vi "tm_sensorcooler_40.vi"(8 "error in (no error)":errorcluster, 10 "Mode":i32(ring)=1 items=["Disable"=1, "Enable"=2], 11 "Handle in":u32) -> (0 "error out":errorcluster, 3 "Handle out":u32)   [LabVIEW 2023]
uses:
  tmcamcon.dll
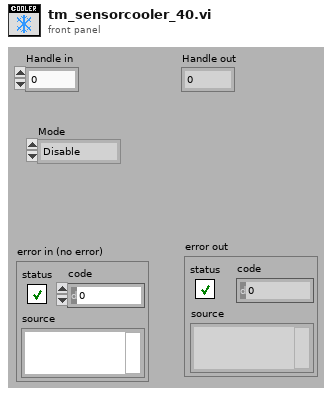
[diagram p1: front panel]
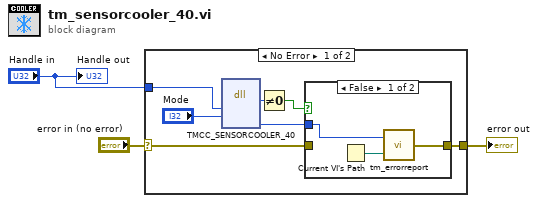
[diagram p0: block diagram]
diagram:
  n1 = case shown="No Error" "error in (no error)" {
    selector: "error in (no error)" -> [w7 w15]
    tunnel: [w4 w15] -> w2
    tunnel: "Handle in" -> [w8 _]
    frame No Error {
      n2 = dll-call lib="tmcamcon.dll" fn="TMCC_SENSORCOOLER_40"("Handle"=w8, "mode"="Mode") -> ("return type"=w10:u32, "Erval"=w5:i32)  [unwired: 6 in, 2 out]
      n3 = Not Equal To 0?(x=w10) -> (x != 0?=w6:bool)
      n4 = case shown="False" w6 {
        tunnel: w7 -> [_ w14]
        tunnel: [w12 w14] -> w4
        tunnel: w5 -> [w11 _]
        frame False {
          n5 = Current VI's Path() -> (path=w13:path)
          n6 = call "tm_errorreport.vi"("Source"=w13, "Error"=w11) -> ("error out"=w12:errorcluster)
        }
        frame True {
        }
      }
    }
    frame Error {
    }
  }
  "error out" <- w2
  "Handle out" <- "Handle in"
